vi "flattenMassToXML_Array.vi"(8 "error in (no error)":errorcluster, 9 "massUnitInXML":T1, 10 "massAgain":variant, 11 "mass":dbl[unit][](array[numeric])) -> (0 "error out":errorcluster, 3 "xmlString":string)   [LabVIEW 2012, in "UnitsAndXML.lvlib"]
uses:
  <userlib>/Common/UnitsAndXML/UnitsAndXML.lvlib
  <userlib>/Common/UnitsAndXML/FlattenItemWithUnitToXML/FlattenMassToXML/MassUnit.ctl
  <vilib>/Utility/VariantDataType/VariantType.lvlib
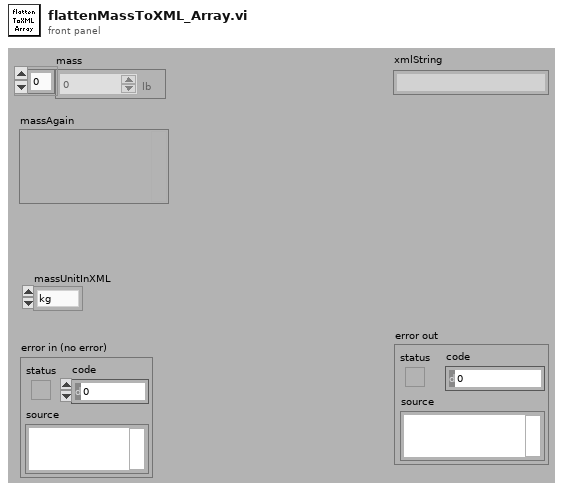
[diagram p1: front panel]
types:
  T1 = typedef "UnitsAndXML.lvlib/MassUnit.ctl" = enum16{"kg", "CM", "dr", "gr", "t", "oz", "lb", "slug", "stone", "Ton", "ton", "u"}
  T2 = typedef "VariantType.lvlib/Type.ctl" = enum8{"Invalid Type", "Void", "I8", "I16", "I32", "I64", "U8", "U16", "U32", "U64", "Single Float", "Double Float", "Extended Float", "Single Complex", "Double Complex", "Extended Complex", "Enum U8", "Enum U16", "Enum U32", "Enum U64", "Single Float With Unit", "Double Float With Unit", "Extended Float With Unit", "Single Complex with Unit", "Double Complex with Unit", "Extended Complex with Unit", "Boolean", "String", "Path", "Picture", "Tag", "Array", "Cluster", "Variant", "LV Variant", "Waveform", "Timestamp", "Digital Waveform", "Digital Data", "ExpressData", "Refnum", "External Data", "VI", "Poly VI", "LabVIEW Class Instance", "Fixed Point"}
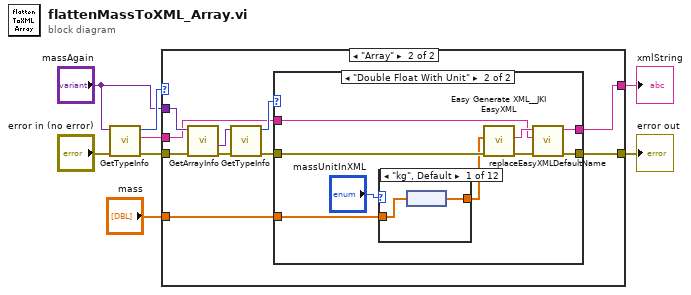
[diagram p0: block diagram]
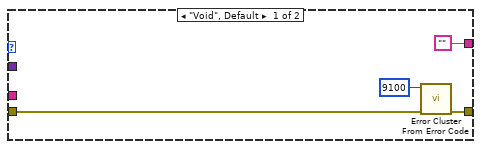
[diagram p2: hidden frame]
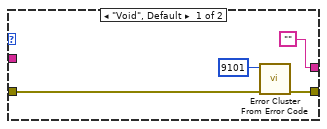
[diagram p3: hidden frame]
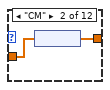
[diagram p4: hidden frame]
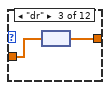
[diagram p5: hidden frame]
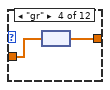
[diagram p6: hidden frame]
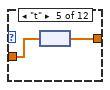
[diagram p7: hidden frame]
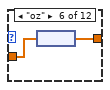
[diagram p8: hidden frame]
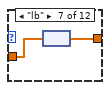
[diagram p9: hidden frame]
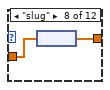
[diagram p10: hidden frame]
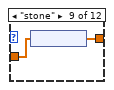
[diagram p11: hidden frame]
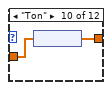
[diagram p12: hidden frame]
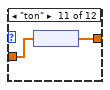
[diagram p13: hidden frame]
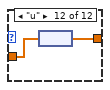
[diagram p14: hidden frame]
diagram:
  n1 = call <vilib>:"GetTypeInfo.vi"("error in (no error)"="error in (no error)", "Variant"="massAgain") -> ("error out"=w2:errorcluster, "Name"=w1:string, "Type Enum"=w4:T2)  [unwired: 5 in, 2 out]
  n2 = case shown="\"Array\"" w4 {
    tunnel: "mass" -> [_ w18]
    tunnel: ["" w16] -> w7
    tunnel: [w9 w17] -> w6
    tunnel: "massAgain" -> [_ w22]
    tunnel: w2 -> [w10 w15]
    tunnel: w1 -> [_ w13]
    frame "Void", Default {
      n3 = call <vilib>:"Error Cluster From Error Code.vi"("error in (no error)"=w10, "error code (0)"=9100) -> ("error out"=w9:errorcluster)  [unwired: 7 in]
    }
    frame "Array" {
      n4 = call <vilib>:"GetArrayInfo.vi"("error in (no error)"=w15, "Variant"=w22) -> ("error out"=w21:errorcluster, "ArrayElement"=w20:variant)  [unwired: 6 in, 2 out]
      n5 = call <vilib>:"GetTypeInfo.vi"("error in (no error)"=w21, "Variant"=w20) -> ("error out"=w14:errorcluster, "Type Enum"=w19:T2)  [unwired: 5 in, 3 out]
      n6 = case shown="\"Double Float With Unit\"" w19 {
        tunnel: w18 -> [_ w28]
        tunnel: ["" w34] -> w16
        tunnel: [w23 w33] -> w17
        tunnel: w14 -> [w24 w32]
        tunnel: w13 -> [_ w30]
        frame "Void", Default {
          n7 = call <vilib>:"Error Cluster From Error Code.vi"("error in (no error)"=w24, "error code (0)"=9101) -> ("error out"=w23:errorcluster)  [unwired: 7 in]
        }
        frame "Double Float With Unit" {
          n8 = case shown="\"kg\", Default" "massUnitInXML" {
            tunnel: [w37 w39 w41 w43 w45 w47 w49 w51 w53 w55 w57 w59] -> w27
            tunnel: w28 -> [w36 w38 w40 w42 w44 w46 w48 w50 w52 w54 w56 w58]
            frame "kg", Default {
              n9 = node(w36) -> (w37:dbl[])
            }
            frame "CM" {
              n10 = node(w38) -> (w39:dbl[])
            }
            frame "dr" {
              n11 = node(w40) -> (w41:dbl[])
            }
            frame "gr" {
              n12 = node(w42) -> (w43:dbl[])
            }
            frame "t" {
              n13 = node(w44) -> (w45:dbl[])
            }
            frame "oz" {
              n14 = node(w46) -> (w47:dbl[])
            }
            frame "lb" {
              n15 = node(w48) -> (w49:dbl[])
            }
            frame "slug" {
              n16 = node(w50) -> (w51:dbl[])
            }
            frame "stone" {
              n17 = node(w52) -> (w53:dbl[])
            }
            frame "Ton" {
              n18 = node(w54) -> (w55:dbl[])
            }
            frame "ton" {
              n19 = node(w56) -> (w57:dbl[])
            }
            frame "u" {
              n20 = node(w58) -> (w59:dbl[])
            }
          }
          n21 = call <vilib>:"Easy Generate XML__JKI EasyXML.vi"("error in (no error)"=w32, "LabVIEW Data"=w27) -> ("error out"=w31:errorcluster, "XML String"=w35:string)  [unwired: 8 in]
          n22 = call <userlib>:"replaceEasyXMLDefaultName.vi"("error in"=w31, "desiredName"=w30, "easyXMLStringWithDefaultNames"=w35) -> ("error out"=w33:errorcluster, "xmlString"=w34:string)  [unwired: 7 in]
        }
      }
    }
  }
  "xmlString" <- w7
  "error out" <- w6
